vi "add function to configuration.vi"(8 "error in":errorcluster, 10 "processing function":T1, 11 "tag bus configurable plugin module configuration in":refnum<class "tag bus processing plugin module configuration.lvclass">) -> (0 "error out":errorcluster, 3 "tag bus configurable plugin module configuration out":refnum<class "tag bus processing plugin module configuration.lvclass">)   [LabVIEW 2013, in "tag bus processing plugin module configuration.lvclass"]
uses:
  tag bus processing plugin module configuration.lvclass
  processing channels.ctl
  <vilib>/NI/Tag Bus Module Framework/channel/TBM channel.lvclass
  <vilib>/NI/Tag Bus/tag/tag descriptor.lvclass/tag descriptor.ctl
  tag bus processing plugin module configuration.lvclass/tag bus processing plugin module configuration.ctl
  <vilib>/NI/Tag Bus/tag/tag descriptor.lvclass
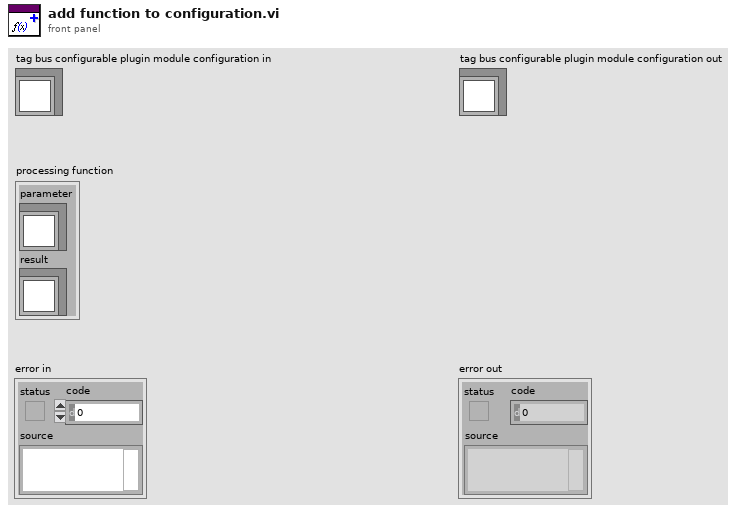
[diagram p1: front panel]
types:
  T1 = typedef "tag bus processing plugin module configuration.lvclass/processing channels.ctl" = cluster{"parameter":refnum<class "TBM channel.lvclass">, "result":refnum<class "TBM channel.lvclass">}
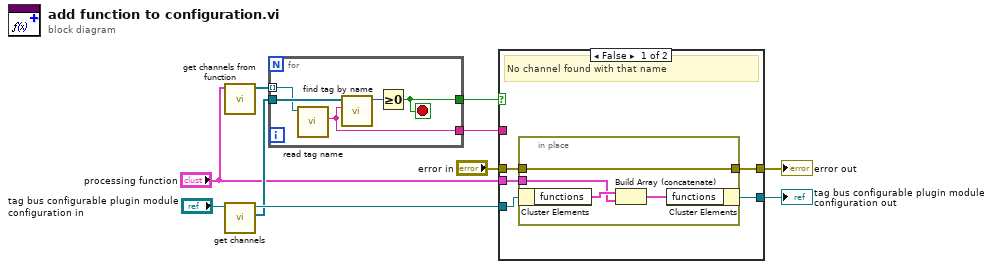
[diagram p0: block diagram]
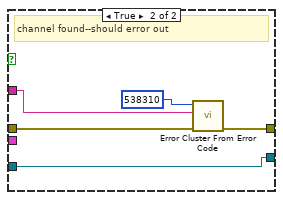
[diagram p2: hidden frame]
diagram:
  n1 = call "get channels from function.vi"("processing function"="processing function") -> ("channels"=w5:refnum<class "TBM channel.lvclass">[])  [unwired: 10 in]
  n2 = call-dynamic "get channels.vi"("module configuration in"="tag bus configurable plugin module configuration in") -> ("channels"=w6:refnum<class "TBM channel.lvclass">[], "module configuration out"=w10:refnum<class "tag bus processing plugin module configuration.lvclass">)  [unwired: 9 in]
  n3 = for {
    tunnel: w6 -> [w15]
    tunnel: w5 -> [w14] mode=indexing
    tunnel: [w12] -> w4
    tunnel: [w11] -> w3
    stop <- w12 stop-if-true
    n4 = call <vilib>:"read tag name.vi"("system tag in"=w14) -> ("name"=w11:string)  [unwired: 8 in, 2 out]
    n5 = call <vilib>:"find tag by name.vi"("name"=w11, "tags in"=w15) -> ("index"=w13:i32)  [unwired: 9 in]
    n6 = Greater Or Equal To 0?(x=w13) -> (x >= 0?=w12:bool)
  }
  n7 = case shown="False" w4 {
    tunnel: [w16 w29] -> w8
    tunnel: w10 -> [w20 w27]
    tunnel: [w19 w27] -> w7
    tunnel: w3 -> [_ w26]
    tunnel: "error in" -> [w17 w25]
    tunnel: "processing function" -> [w18 _]
    frame False {
      # "No channel found with that name"
      n8 = in-place {
        in-place-border: w18 -> [w23]
        in-place-border: w17 -> [w21]
        in-place-border: [w21] -> w16
        n9 = in-place-cluster #1(w20) -> ("functions"=w24:T1[])
        n10 = Build Array (concatenate)(w24, w23) -> (w22:T1[])
        n11 = in-place-cluster #1("functions"=w22) -> (w19:refnum<class "tag bus processing plugin module configuration.lvclass">)
      }
    }
    frame True {
      # "channel found--should error out"
      n12 = call <vilib>:"Error Cluster From Error Code.vi"("error in (no error)"=w25, "error message (\"\")"=w26, "error code (0)"=538310) -> ("error out"=w29:errorcluster)  [unwired: 6 in]
    }
  }
  "error out" <- w8
  "tag bus configurable plugin module configuration out" <- w7
